vi "Set All Channels.vi"(8 "error in (no error)":errorcluster, 10 "allChannelProperties":T1 {"channel" min=1 max=8 step=1}, 11 "VISA Refnum in":refnum<visa-resource-name>="COM1") -> (0 "error out":errorcluster, 2 "allChannelProperties":T1 {"channel" min=1 max=8 step=1}, 3 "VISA Refnum out":refnum<visa-resource-name>)   [LabVIEW 2019, in "KH7008.lvlib"]
uses:
  KH7008.lvlib
  typedefs/allChannelProperties--Array.ctl
  typedefs/channelProperties--Cluster.ctl
  typedefs/channel--numeric.ctl
  typedefs/gain--enum.ctl
  typedefs/Input--Enum.ctl
  typedefs/shunt--enum.ctl
  typedefs/couple--Enum.ctl
  typedefs/Filter--Enum.ctl
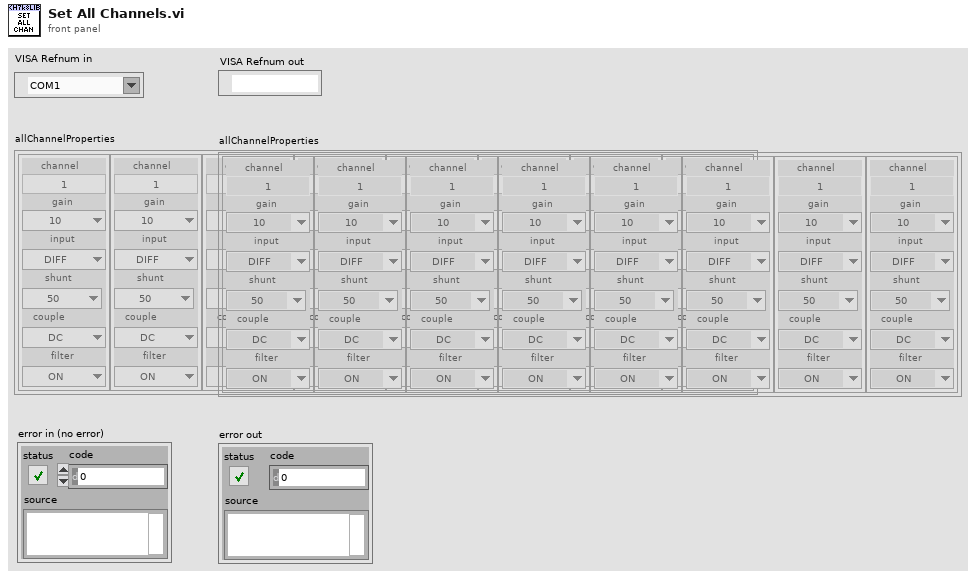
[diagram p1: front panel]
types:
  T1 = typedef "KH7008.lvlib/allChannelProperties--Array.ctl" = T2[]
  T2 = typedef "KH7008.lvlib/channelProperties--Cluster.ctl" = cluster{"channel":T3, "gain":T4, "input":T5, "shunt":T6, "couple":T7, "filter":T8}
  T3 = typedef "KH7008.lvlib/channel--numeric.ctl" = u16
  T4 = typedef "KH7008.lvlib/gain--enum.ctl" = enum16{"1", "10", "100", "1000"}
  T5 = typedef "KH7008.lvlib/input--enum.ctl" = enum16{"OFF", "SE+", "SE-", "DIFF"}
  T6 = typedef "KH7008.lvlib/shunt--enum.ctl" = enum16{"Open", "50", "500", "5k", "50k", "10M"}
  T7 = typedef "KH7008.lvlib/couple--enum.ctl" = enum16{"AC", "DC"}
  T8 = typedef "KH7008.lvlib/filter--enum.ctl" = enum16{"OFF", "ON"}
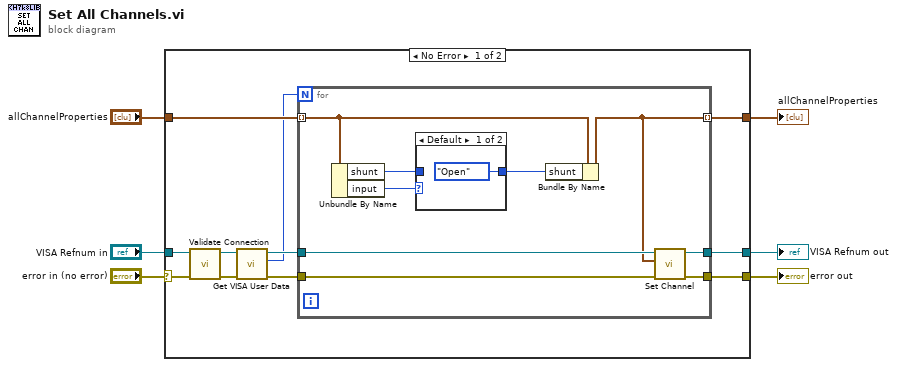
[diagram p0: block diagram]
diagram:
  n1 = case shown="No Error" "error in (no error)" {
    selector: "error in (no error)" -> [w13 w31]
    tunnel: "allChannelProperties" -> [w17 w29]
    tunnel: "VISA Refnum in" -> [w12 w30]
    tunnel: [w16 w31] -> w4
    tunnel: [w15 w30] -> w2
    tunnel: [w14 w29] -> w1
    frame No Error {
      n2 = call "Validate Connection.vi"("error in (no error)"=w13, "VISA Refnum in"=w12) -> ("error out"=w8:errorcluster, "VISA Refnum out"=w9:refnum<visa-resource-name>)  [unwired: 8 in]
      n3 = call "Get VISA User Data.vi"("error in (no error)"=w8, "VISA Refnum in"=w9) -> ("error out"=w11:errorcluster, "User Data"=w7:i32, "VISA Refnum out"=w10:refnum<visa-resource-name>)  [unwired: 7 in]
      n4 = for {
        N: w7 -> [_]
        tunnel: w17 -> [w20] mode=indexing
        tunnel: [w18] -> w14 mode=indexing
        tunnel: w10 -> [w25]
        tunnel: [w19] -> w15
        tunnel: w11 -> [w22]
        tunnel: [w26] -> w16
        n5 = Unbundle By Name(w20) -> ("shunt"=w24:T6, "input"=w23:T5)
        n6 = case shown="Default" w23 {
          tunnel: [shunt--enum."Open" ("f") w28] -> w21
          tunnel: w24 -> [_ w28]
          frame Default {
          }
          frame "DIFF" {
          }
        }
        n7 = Bundle By Name(cluster=w20, "shunt"=w21) -> (w18:T2)
        n8 = call "Set Channel.vi"("error in (no error)"=w22, "channelParameter"=w18, "VISA Refnum in"=w25) -> ("error out"=w26:errorcluster, "VISA Refnum out"=w19:refnum<visa-resource-name>)  [unwired: 7 in]
      }
    }
    frame Error {
    }
  }
  "error out" <- w4
  "VISA Refnum out" <- w2
  "allChannelProperties" <- w1
